vi "Stop Core.vi"(10 "final error code":i32, 11 "IViewModel in":refnum<class "IViewModel.lvclass">) -> (3 "IViewModel out":refnum<class "IViewModel.lvclass">)   [LabVIEW 2019, in "IViewModel.lvlib" / "IViewModel.lvclass"]
doc: "(<B>Filename</B>: Actor Framework.lvlib:Actor.lvclass:Stop Core.vi)\n\nDefines what the actor does before it stops. Use the <B>final error code</B> input to determine whether the actor shut down in response to an error.\n\nBy default, this method does nothing. A descendant class may override it to define behavior, such as shutting down any processes the actor initiated in its override of the Actor Core method.\n\n<License>\nCopyright © 2017 Composed Systems, LLC | All rights reserved\nwww.composed.io\n\nAuthor: Ethan Stern <ethan.stern@composed.io>\n\nThis software is provided \"AS IS\" WITHOUT WARRANTIES, either express or implied, AND IS FOR EDUCATIONAL PURPOSES ONLY.\n</License>"
uses:
  <vilib>/gpm_packages/@cs/mva-viewable/Source/IViewModel/IViewModel/IViewModel.lvclass
  C:/Program Files/National Instruments/LabVIEW 2019/vi.lib/gpm_packages/@cs/mva-core/Source/IObserver/IObserver/IObserver.lvclass
  <vilib>/gpm_packages/@cs/mva-viewable/Source/IViewModel/IViewModel/IViewModel.lvclass/IViewModel.ctl
  <vilib>/gpm_packages/@cs/event-logger/Source/Composed Log/Types/Log Level.ctl
  <vilib>/gpm_packages/@cs/mva-core/Source/IObserver/IObserver/IObserver.lvclass/IObserver.ctl
  <vilib>/gpm_packages/@cs/event-logger/Source/Composed Log/LoggerReference/LoggerReference.lvclass/LoggerReference.ctl
  <vilib>/ActorFramework/Message Enqueuer/Message Enqueuer.lvclass/Message Enqueuer.ctl
  <vilib>/gpm_packages/@cs/event-logger/Source/Composed Log/LoggerReference/Log Event.vi
  <vilib>/ActorFramework/Message Enqueuer/Enqueue.vi
  <vilib>/gpm_packages/@cs/event-logger/Source/Composed Log/LoggerReference/Log.vi
  <vilib>/gpm_packages/@cs/event-logger/Source/Composed Log/LoggerReference/Get Valid Event Time.vi
  <vilib>/gpm_packages/@cs/event-logger/Source/Composed Log/LoggerReference/Remove Stale Logs.vi
  <vilib>/ActorFramework/Stop Msg/Stop Msg.lvclass
  C:/Program Files/National Instruments/LabVIEW 2019/vi.lib/ActorFramework/Message/Message.lvclass
  <vilib>/Utility/LVClass/Get LV Class Name.vi
  <vilib>/gpm_packages/@cs/event-logger/Source/Composed Log/LoggerReference/Close Local Event Log.vi
  <vilib>/ActorFramework/Message Priority Queue/Priority Enqueue.vi
  <vilib>/gpm_packages/@cs/mva-viewable/Source/IViewManager/IViewManager/IViewManager.lvclass
  <vilib>/gpm_packages/@cs/mva-viewable/Source/IViewable/ProtectedSubpanel/ProtectedSubpanel.lvclass
  <vilib>/gpm_packages/@cs/mva-core/Source/IObserver/IObserver/IObserver.lvclass
  <vilib>/gpm_packages/@cs/event-logger/Source/Composed Log/Composed Log.lvlib
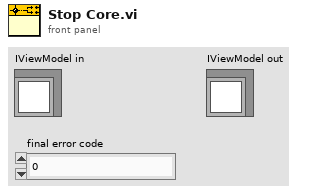
[diagram p1: front panel]
types:
  T1 = typedef "IViewable.lvlib/ProtectedSubpanel.lvclass/Protected Subpanel Reference.ctl" = refnum<data-value>
  T2 = typedef "Composed Log.lvlib/Log Level.ctl" = enum16{"Debug", "Info", "Warning", "Error", "Critical"}
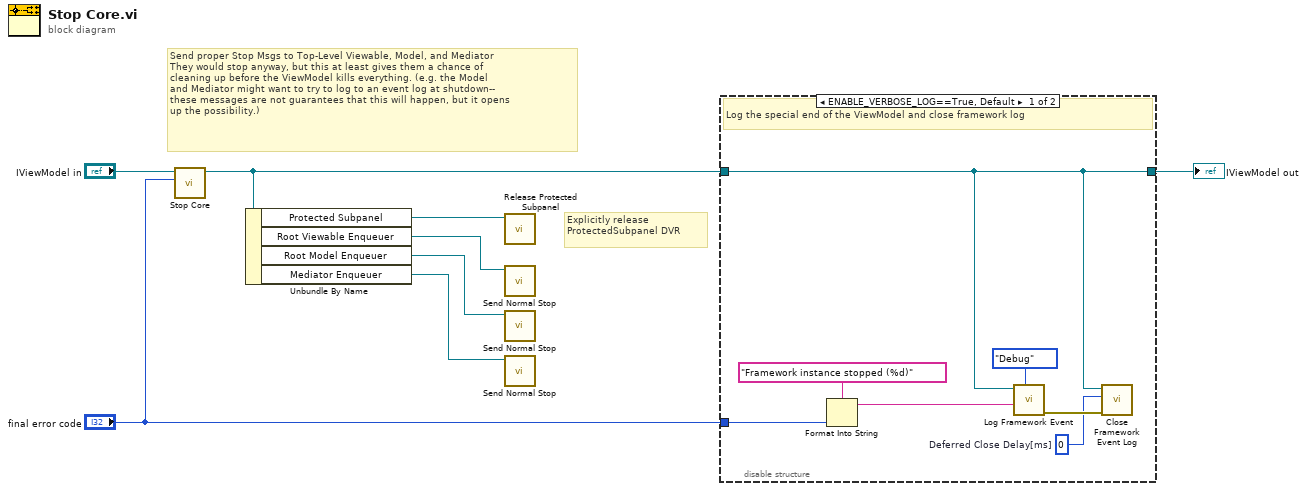
[diagram p0: block diagram]
diagram:
  # "Explicitly release\nProtectedSubpanel DVR"
  # "Send proper Stop Msgs to Top-Level Viewable, Model, and Mediator\nThey would stop anyway, but this at least gives them a chance of\ncleaning up before the ViewModel kills everything. (e.g. the Model\nand Mediator might want to try to log to an event log at shutdown--\nthese messages are not guarantees that this will happen, but it opens\nup the possibility.)"
  n1 = call-parent "Stop Core.vi"("final error code"="final error code", "IViewManager in"="IViewModel in") -> ("IViewManager out"=w3:refnum<class "IViewModel.lvclass">)  [unwired: 9 in]
  n2 = Unbundle By Name(w3) -> ("Protected Subpanel"=w4:T1, "Root Viewable Enqueuer"=w5:refnum<class "Message Enqueuer.lvclass">, "Root Model Enqueuer"=w7:refnum<class "Message Enqueuer.lvclass">, "Mediator Enqueuer"=w6:refnum<class "Message Enqueuer.lvclass">)
  n3 = call <vilib>:"Release Protected Subpanel.vi"("Protected Subpanel"=w4) -> ()  [unwired: 10 in, 1 out]
  n4 = call <vilib>:"Send Normal Stop.vi"("Message Enqueuer"=w5) -> ()  [unwired: 10 in, 1 out]
  n5 = call <vilib>:"Send Normal Stop.vi"("Message Enqueuer"=w7) -> ()  [unwired: 10 in, 1 out]
  n6 = call <vilib>:"Send Normal Stop.vi"("Message Enqueuer"=w6) -> ()  [unwired: 10 in, 1 out]
  n7 = disable-structure shown="ENABLE_VERBOSE_LOG==True, Default" {
    disable-tunnel: w3 -> [w10 w16]
    disable-tunnel: [w10 w16] -> w2
    disable-tunnel: "final error code" -> [w14 _]
    frame condition #0 (active) {
      w9 = u32 0  # Deferred Close Delay[ms]
      # "Log the special end of the ViewModel and close framework log"
      n8 = Format Into String(format string="Framework instance stopped (%d)", w14) -> (resulting string=w12:string)  [unwired: 2 in, 1 out]
      n9 = call <vilib>:"Log Framework Event.vi"("Event Level (Debug)"=Log_Level."Debug" ("Event Level"), "Data To Log"=w12, "IObserver in"=w10) -> ("error out"=w11:errorcluster)  [unwired: 8 in]
      n10 = call <vilib>:"Close Framework Event Log.vi"("error in (no error)"=w11, "Deferred Close Time (0 ms)"=w9, "IObserver in"=w10) -> ()  [unwired: 9 in]
    }
    frame condition #1 {
      # "Remove all logging from this method at compile time"
    }
  }
  "IViewModel out" <- w2
